vi "ReadFromPTC10_Old.vi"(8 "error in (no error)":errorcluster, 11 "VISA Refnum in":refnum<visa-resource-name>) -> (0 "error out":errorcluster, 1 "relays":i8=4, 2 "Cycles":i16, 3 "Temperature Chart":T1(graph), 4 "Heater Output":dbl, 5 "Target Temperature":dbl)   [LabVIEW 2023]
uses:
  <vilib>/Instr/_visa.llb/VISA Flush IO Buffer Mask.ctl
  <instrlib>/Stanford PTC10/SRS PTC10.lvlib
panel:
  out "Output as text":string
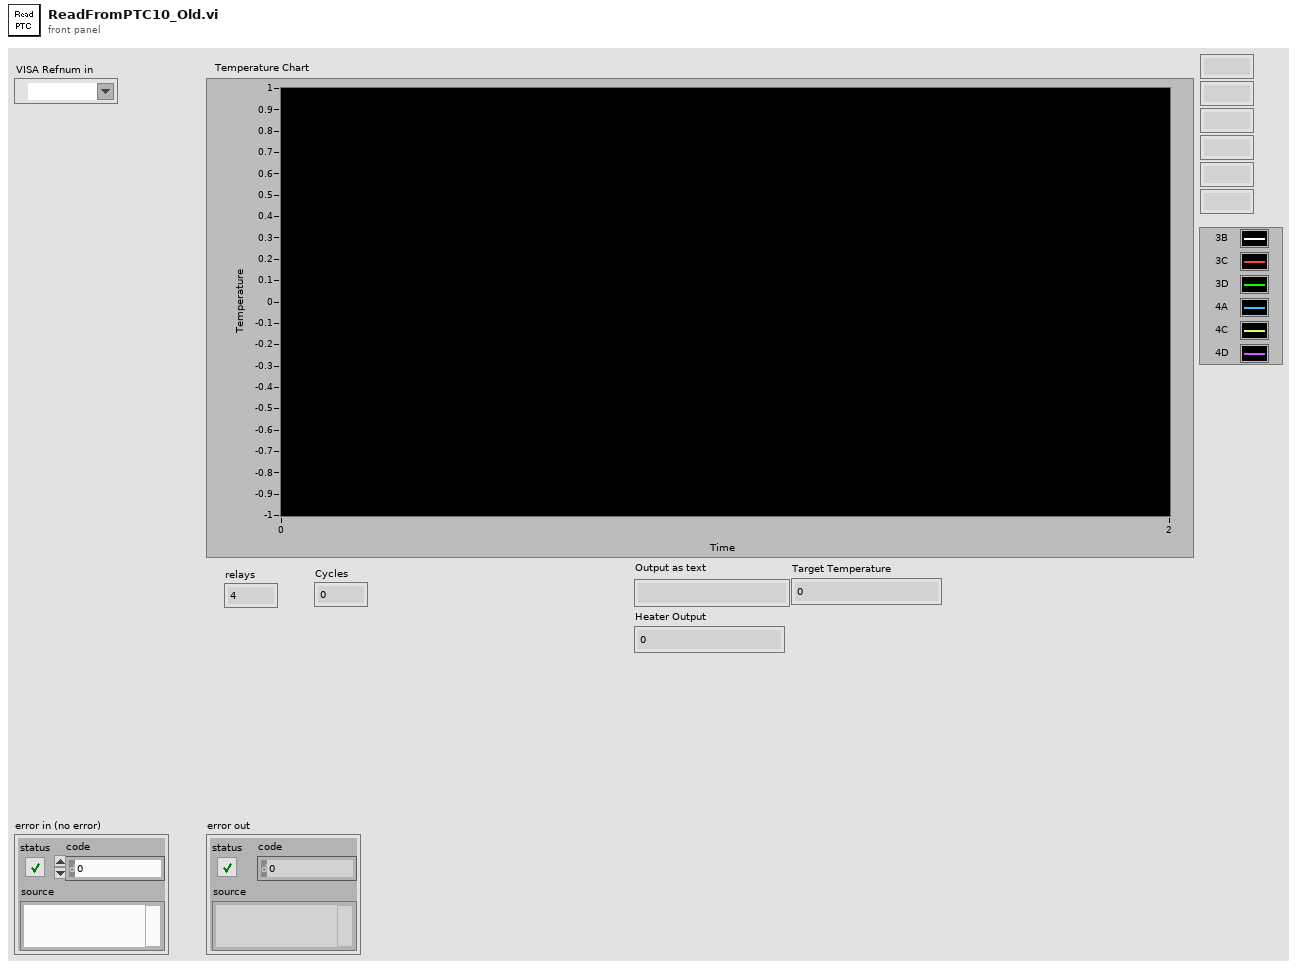
[diagram p1: front panel]
types:
  T1 = cluster{"Output as number":dbl, "Output as number":dbl, "Output as number":dbl, "Output as number":dbl, "Output as number":dbl, "Output as number":dbl}
  T2 = typedef "VISA Flush IO Buffer Mask.ctl" = u16
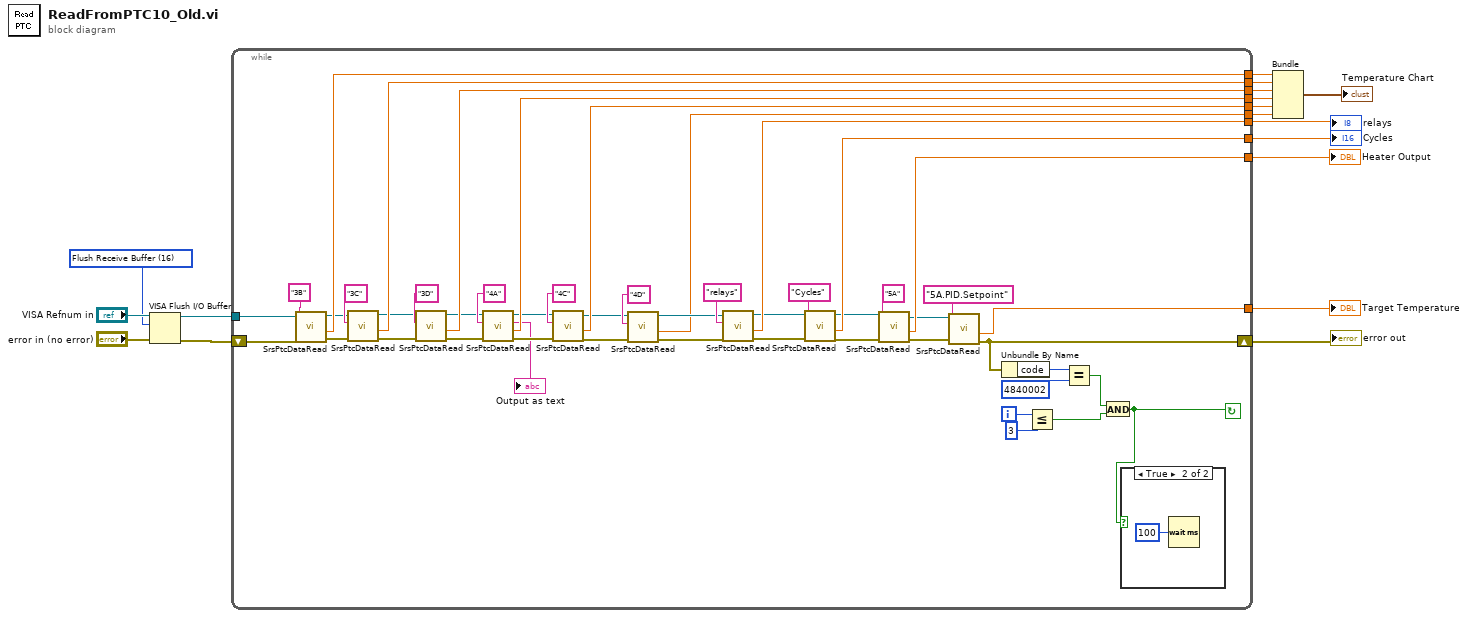
[diagram p0: block diagram]
diagram:
  w6 = T2 16 items=["Flush Receive Buffer"=16, "Write Transmit Buffer to Device"=32, "Flush Receive Buffer (No I/O)"=64, "Flush Transmit Buffer"=128] ("Mask")
  n1 = VISA Flush I/O Buffer(VISA resource name="VISA Refnum in", mask (16)=w6, error in (no error)="error in (no error)") -> (VISA resource name out=w7:refnum<visa-resource-name>, error out=w9:errorcluster)
  n2 = while {
    tunnel: [w65] -> w16
    tunnel: [w64] -> w15
    tunnel: [w63] -> w14
    tunnel: [w55] -> w13
    tunnel: [w53] -> w12
    tunnel: [w47] -> w11
    tunnel: w7 -> [w45]
    tunnel: [w41] -> w5
    tunnel: [w37] -> w3
    tunnel: [w34] -> w2
    shift-right: [w31] -> w4
    shift-left: w9 -> [w46]
    tunnel: [w18] -> w1
    i -> [w28]
    stop <- w24 continue-if-true
    n3 = call <instrlib>:"SrsPtcDataRead.vi"("error in"=w46, "Channel"="3B", "SRS PTC10 VISA in"=w45) -> ("error out"=w59:errorcluster, "Output as number"=w63:dbl, "SRS PTC10 VISA out"=w57:refnum<visa-resource-name>)  [unwired: 5 in, 1 out]
    n4 = call <instrlib>:"SrsPtcDataRead.vi"("error in"=w59, "Channel"="3C", "SRS PTC10 VISA in"=w57) -> ("error out"=w60:errorcluster, "Output as number"=w64:dbl, "SRS PTC10 VISA out"=w58:refnum<visa-resource-name>)  [unwired: 5 in, 1 out]
    n5 = call <instrlib>:"SrsPtcDataRead.vi"("error in"=w60, "Channel"="3D", "SRS PTC10 VISA in"=w58) -> ("error out"=w52:errorcluster, "Output as number"=w65:dbl, "SRS PTC10 VISA out"=w51:refnum<visa-resource-name>)  [unwired: 5 in, 1 out]
    n6 = call <instrlib>:"SrsPtcDataRead.vi"("error in"=w52, "Channel"="4A", "SRS PTC10 VISA in"=w51) -> ("error out"=w35:errorcluster, "Output as number"=w53:dbl, "Output as text"=→"Output as text":string, "SRS PTC10 VISA out"=w33:refnum<visa-resource-name>)  [unwired: 5 in]
    n7 = call <instrlib>:"SrsPtcDataRead.vi"("error in"=w35, "Channel"="4C", "SRS PTC10 VISA in"=w33) -> ("error out"=w20:errorcluster, "Output as number"=w34:dbl, "SRS PTC10 VISA out"=w22:refnum<visa-resource-name>)  [unwired: 5 in, 1 out]
    n8 = call <instrlib>:"SrsPtcDataRead.vi"("error in"=w20, "Channel"="4D", "SRS PTC10 VISA in"=w22) -> ("error out"=w19:errorcluster, "Output as number"=w18:dbl, "SRS PTC10 VISA out"=w21:refnum<visa-resource-name>)  [unwired: 5 in, 1 out]
    n9 = call <instrlib>:"SrsPtcDataRead.vi"("error in"=w19, "Channel"="relays", "SRS PTC10 VISA in"=w21) -> ("error out"=w50:errorcluster, "Output as number"=w55:dbl, "SRS PTC10 VISA out"=w49:refnum<visa-resource-name>)  [unwired: 5 in, 1 out]
    n10 = call <instrlib>:"SrsPtcDataRead.vi"("error in"=w50, "Channel"="Cycles", "SRS PTC10 VISA in"=w49) -> ("error out"=w43:errorcluster, "Output as number"=w47:dbl, "SRS PTC10 VISA out"=w42:refnum<visa-resource-name>)  [unwired: 5 in, 1 out]
    n11 = call <instrlib>:"SrsPtcDataRead.vi"("error in"=w43, "Channel"="5A", "SRS PTC10 VISA in"=w42) -> ("error out"=w39:errorcluster, "Output as number"=w41:dbl, "SRS PTC10 VISA out"=w38:refnum<visa-resource-name>)  [unwired: 5 in, 1 out]
    n12 = call <instrlib>:"SrsPtcDataRead.vi"("error in"=w39, "Channel"="5A.PID.Setpoint", "SRS PTC10 VISA in"=w38) -> ("error out"=w31:errorcluster, "Output as number"=w37:dbl)  [unwired: 5 in, 2 out]
    n13 = Unbundle By Name(w31) -> ("code"=w30:i32)
    n14 = Less Or Equal?(x=w28, y=3) -> (x <= y?=w25:bool)
    n15 = Equal?(x=w30, y=4840002) -> (x = y?=w26:bool)
    n16 = And(x=w26, y=w25) -> (x .and. y?=w24:bool)
    n17 = case shown="True" w24 {
      frame False {
      }
      frame True {
        n18 = Wait (ms)(milliseconds to wait=u32 100 ("millisecond multiple")) -> ()  [unwired: 1 out]
      }
    }
  }
  "relays" <- w13
  "error out" <- w4
  "Cycles" <- w11
  "Heater Output" <- w5
  "Target Temperature" <- w3
  n19 = Bundle("Output as number"=w14, "Output as number"=w15, "Output as number"=w16, "Output as number"=w12, "Output as number"=w2, "Output as number"=w1) -> (→"Temperature Chart":T1)  [unwired: 1 in]
